vi "solar_misc Elapsed Time.vi"(2 "Reset? (F)":bool, 4 "Time Target (500ms)":u32=500, 8 "error in (no error)":errorcluster) -> (1 "Elapsed?":bool, 5 "error out":errorcluster, 7 "Elapsed Time (s)":u32)   [LabVIEW 2018]
doc: "This returns true if the time target has elapsed."
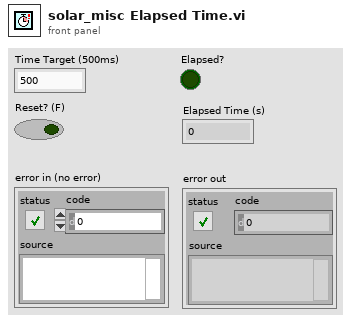
[diagram p1: front panel]
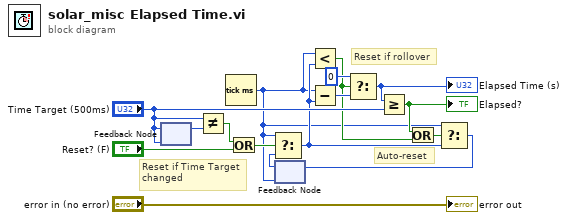
[diagram p0: block diagram]
diagram:
  # "Reset if rollover"
  # "Auto-reset"
  # "Reset if Time Target\nchanged"
  n1 = feedback #1("Time Target (500ms)") -> (w12:u32)
  n2 = feedback-in #1("Time Target (500ms)") -> ()
  n3 = Not Equal?(x="Time Target (500ms)", y=w12) -> (x != y?=w10:bool)
  n4 = Tick Count (ms)() -> (millisecond timer value=w1:u32)
  n5 = Or(x=w10, y="Reset? (F)") -> (x .or. y?=w11:bool)
  n6 = feedback #2(w1) -> (w9:u32)
  n7 = Select(t=w1, s=w11, f=w9) -> (s? t:f=w3:u32)
  n8 = Less?(x=w1, y=w3) -> (x < y?=w2:bool)
  n9 = Subtract(x=w1, y=w3) -> (x-y=w6:u32)
  n10 = Select(t=u32 0, s=w2, f=w6) -> (s? t:f=w5:u32)
  "Elapsed Time (s)" <- w5
  n11 = Greater Or Equal?(x=w5, y="Time Target (500ms)") -> (x >= y?=w15:bool)
  "Elapsed?" <- w15
  n12 = Or(x=w15, y=w2) -> (x .or. y?=w4:bool)
  n13 = Select(t=w1, s=w4, f=w3) -> (s? t:f=w16:u32)
  n14 = feedback-in #2(w16) -> ()
  "error out" <- "error in (no error)"
